vi "VISA Serial Break (Instr).vi"(3 "error in (no error)":errorcluster, 4 "Duration (-1 : use default)":i16=-1, 5 "VISA resource name":refnum<visa-resource-name>) -> (0 "error out":errorcluster, 2 "VISA resource name out":refnum<visa-resource-name>)   [LabVIEW 2020]
doc: "Sends a break on the specified output port. Wire data to the <B>VISA resource name</B> input to determine the polymorphic instance to use or manually select the instance."
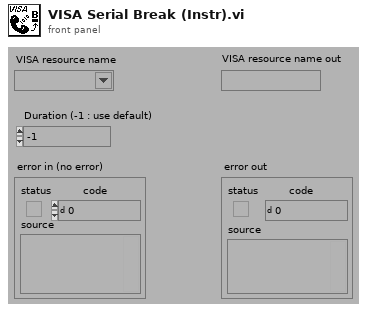
[diagram p1: front panel]
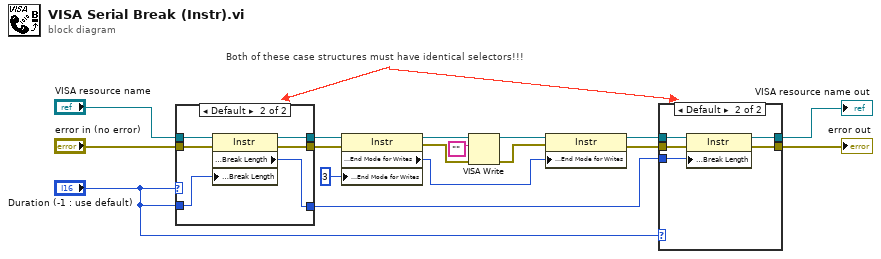
[diagram p0: block diagram]
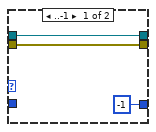
[diagram p3: hidden frame]
diagram:
  # "Both of these case structures must have identical selectors!!!"
  n1 = case shown="Default" "Duration (-1 : use default)" {
    tunnel: "VISA resource name" -> [w20 w26]
    tunnel: "error in (no error)" -> [w19 w25]
    tunnel: [w19 w24] -> w13
    tunnel: [w20 w23] -> w14
    tunnel: [i16 -1 ("Break Len") w22] -> w17
    tunnel: "Duration (-1 : use default)" -> [_ w21]
    frame ..-1 {
    }
    frame Default {
      n2 = property class="Instr"(reference=w26, error in=w25, "Serial Settings:Break Length"=w21) -> (reference out=w23:refnum<visa-resource-name>, error out=w24:errorcluster, "Serial Settings:Break Length"=w22:i16)
    }
  }
  n3 = property class="Instr"(reference=w14, error in=w13, "Serial Settings:End Mode for Writes"=u16 3 ("ASRL End Out")) -> (reference out=w8:refnum<visa-resource-name>, error out=w10:errorcluster, "Serial Settings:End Mode for Writes"=w7:u16)
  n4 = VISA Write(VISA resource name=w8, write buffer="", error in (no error)=w10) -> (VISA resource name out=w9:refnum<visa-resource-name>, error out=w11:errorcluster)  [unwired: 1 out]
  n5 = property class="Instr"(reference=w9, error in=w11, "Serial Settings:End Mode for Writes"=w7) -> (reference out=w15:refnum<visa-resource-name>, error out=w16:errorcluster)
  n6 = case shown="Default" "Duration (-1 : use default)" {
    tunnel: w15 -> [w28 w33]
    tunnel: w16 -> [w27 w32]
    tunnel: [w27 w31] -> w1
    tunnel: [w28 w30] -> w2
    tunnel: w17 -> [_ w29]
    frame ..-1 {
    }
    frame Default {
      n7 = property class="Instr"(reference=w33, error in=w32, "Serial Settings:Break Length"=w29) -> (reference out=w30:refnum<visa-resource-name>, error out=w31:errorcluster)
    }
  }
  "VISA resource name out" <- w2
  "error out" <- w1
